vi "Send Command.vi"(0 "Session Handle in":T1, 5 "REx Command in":refnum<class "REx Command - Root.lvclass">, 11 "error in (no error)":errorcluster) -> (4 "Session Handle out":T1, 6 "REx Command out":refnum<class "REx Command - Root.lvclass">, 15 "error out":errorcluster)   [LabVIEW 2012, in "REx.lvlib" / "Remote Connection Session.lvclass"]
uses:
  Remote Connection Session.lvclass
  Typedefs/Session Handle.ctl
  REx Command Root/REx Command - Root.lvclass
  Remote Connection Session.lvclass/Remote Connection Session.ctl
  Local Listener Session/EXPORT - Invoke Command.vi
  Local Listener Session/Local Listener Session.lvclass
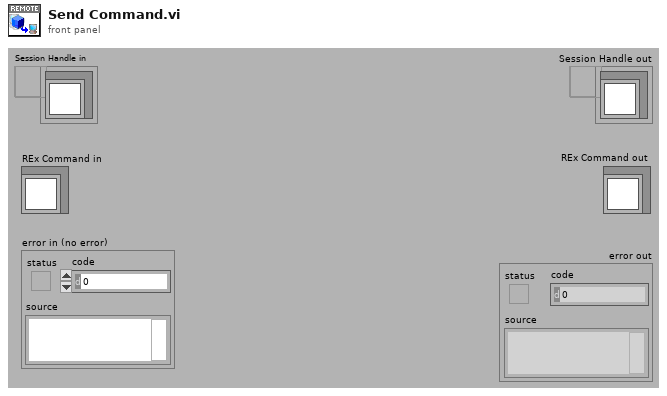
[diagram p1: front panel]
types:
  T1 = typedef "REx.lvlib/Remote Connection Session.lvclass/Session Handle.ctl" = refnum<data-value>
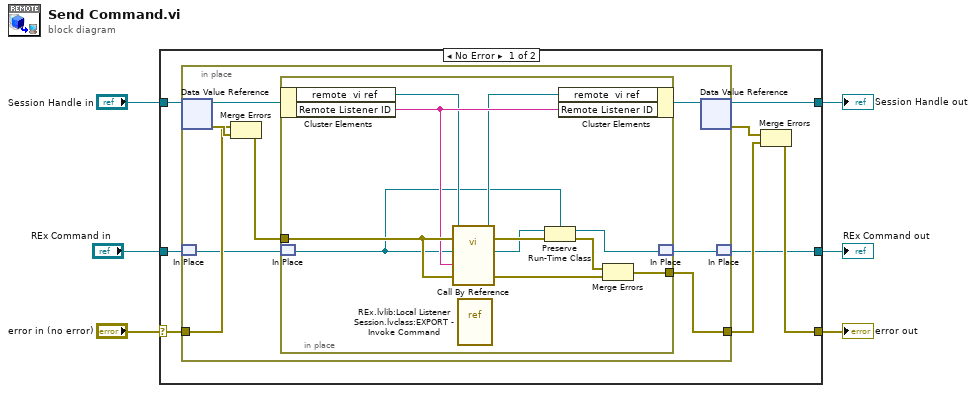
[diagram p0: block diagram]
diagram:
  n1 = case shown="No Error" "error in (no error)" {
    selector: "error in (no error)" -> [w10 w35]
    tunnel: "Session Handle in" -> [w14 w36]
    tunnel: [w13 w36] -> w5
    tunnel: [w11 w35] -> w4
    tunnel: "REx Command in" -> [w8 w34]
    tunnel: [w7 w34] -> w1
    frame No Error {
      n2 = in-place {
        in-place-border: w10 -> [w20]
        in-place-border: [w19] -> w9
        n3 = in-place-dvr #1(w14) -> (w18:refnum<class "Remote Connection Session.lvclass">, w21:errorcluster)
        n4 = in-place-match #2(w8) -> (w16:refnum<class "REx Command - Root.lvclass">)
        n5 = Merge Errors(w20, w21) -> (w22:errorcluster)
        n6 = in-place {
          in-place-border: w22 -> [w32]
          in-place-border: [w28] -> w19
          n7 = in-place-cluster #3(w18) -> ("remote  vi ref"=w26:refnum<vi>, "Remote Listener ID"=w27:string)
          n8 = in-place-match #4(w16) -> (w24:refnum<class "REx Command - Root.lvclass">)
          n9 = call-by-ref "?"(reference=w26, error in=w32, "REx.lvlib:REx Command - Root.lvclass"=w24, "Session ID"=w27, 11:"error in (no error)"=w32) -> (reference out=w25:refnum<vi>, error out=w33:errorcluster, "REx.lvlib:REx Command - Root.lvclass"=w30:refnum<class "REx Command - Root.lvclass">, 15:"error out"=w31:errorcluster)  [unwired: 11 in]
          n10 = vi-ref "REx.lvlib:Local Listener Session.lvclass:EXPORT - Invoke Command.vi"() -> ()  [unwired: 1 out]
          n11 = Preserve Run-Time Class(object in=w30, error in=w33, 2:w24) -> (object out=w23:refnum<class "REx Command - Root.lvclass">, error out=w29:errorcluster)
          n12 = in-place-cluster #3("remote  vi ref"=w25, "Remote Listener ID"=w27) -> (w17:refnum<class "Remote Connection Session.lvclass">)
          n13 = Merge Errors(w29, w31) -> (w28:errorcluster)
          n14 = in-place-match #4(w23) -> (w15:refnum<class "REx Command - Root.lvclass">)
        }
        n15 = in-place-dvr #1(w17) -> (w13:T1, w12:errorcluster)
        n16 = in-place-match #2(w15) -> (w7:refnum<class "REx Command - Root.lvclass">)
      }
      n17 = Merge Errors(w12, w9) -> (w11:errorcluster)
    }
    frame Error {
    }
  }
  "Session Handle out" <- w5
  "error out" <- w4
  "REx Command out" <- w1
